vi "error modelling.vi"(10 "Frequency":dbl=200.0, 11 "Gyroscope":dbl[](array[numeric])) -> (1 "actual sample time (s)":dbl)   [LabVIEW 2021]
uses:
  <vilib>/Utility/error.llb/DialogType.ctl
panel:
  out "Allan Variance":dbl
  in  "n":i32
  out "error out 2":errorcluster
  in  "error in (no error) 2":errorcluster
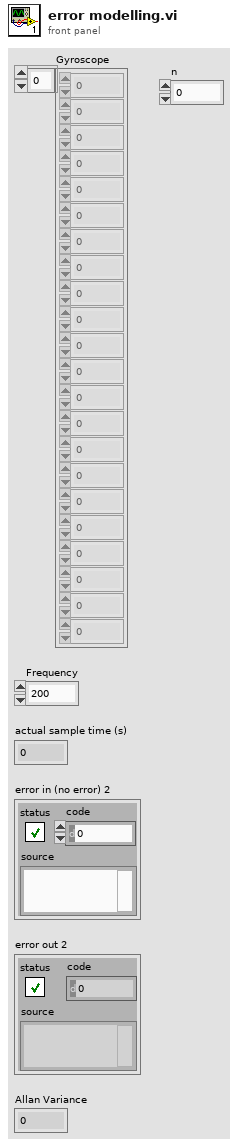
[diagram p1: front panel]
types:
  T1 = typedef "DialogType.ctl" = u16
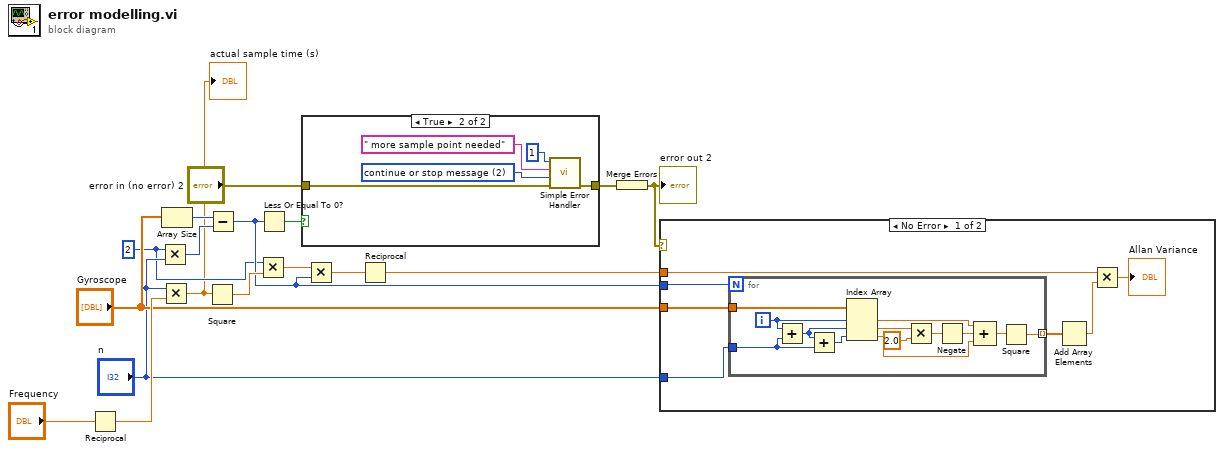
[diagram p0: block diagram]
diagram:
  w3 = 2 ("x")
  n1 = Reciprocal(x="Frequency") -> (1/x=w12:dbl)
  n2 = Multiply(x=w3, y="n") -> (x*y=w10:i32)
  n3 = Multiply(x="n", y=w12) -> (x*y=w1:dbl)
  "actual sample time (s)" <- w1
  n4 = Array Size(array="Gyroscope") -> (size(s)=w11:i32)
  n5 = Square(x=w1) -> (x^2=w9:dbl)
  n6 = Subtract(x=w11, y=w10) -> (x-y=w7:i32)
  n7 = Multiply(x=w3, y=w9) -> (x*y=w8:dbl)
  n8 = Less Or Equal To 0?(x=w7) -> (x <= 0?=w17:bool)
  n9 = case shown="True" w17 {
    tunnel: "error in (no error) 2" -> [w18 w23]
    tunnel: [w18 w22] -> w16
    frame False {
    }
    frame True {
      w20 = T1 2 items=["no dialog", "OK message", "continue or stop message", "OK message + warnings", "continue/stop + warnings"] ("type of dialog (OK msg:1)")
      n10 = call <vilib>:"Simple Error Handler.vi"("error code (no error:0)"=1, "error source (\" \")"=" more sample point needed" ("error source (\" \")"), "type of dialog (OK msg:1)"=w20, "error in (no error)"=w23) -> ("error out"=w22:errorcluster)  [unwired: 1 in, 4 out]
    }
  }
  n11 = Multiply(x=w8, y=w7) -> (x*y=w6:dbl)
  n12 = Reciprocal(x=w6) -> (1/x=w2:dbl)
  n13 = Merge Errors(w16) -> (w14:errorcluster)
  "error out 2" <- w14
  n14 = case shown="No Error" w14 {
    tunnel: w7 -> [w30 _]
    tunnel: "Gyroscope" -> [w29 _]
    tunnel: "n" -> [w28 _]
    tunnel: w2 -> [w25 _]
    frame No Error {
      n15 = for {
        N: w30 -> [_]
        tunnel: w29 -> [w38]
        tunnel: w28 -> [w40]
        tunnel: [w31] -> w27 mode=indexing
        i -> [w41]
        n16 = Add(x=w41, y=w40) -> (x+y=w42:i32)
        n17 = Add(x=w42, y=w40) -> (x+y=w43:i32)
        n18 = Index Array(array=w38, index #1=w41, index #2=w42, index #3=w43) -> (element #1=w39:dbl, element #2=w37:dbl, element #3=w36:dbl)
        n19 = Multiply(x=w37, y=2.0) -> (x*y=w35:dbl)
        n20 = Negate(x=w35) -> (-x=w33:dbl)
        n21 = Compound Arithmetic op=ADD(w39, w33, w36) -> (w32:dbl)
        n22 = Square(x=w32) -> (x^2=w31:dbl)
      }
      n23 = Add Array Elements(numeric array=w27) -> (sum=w26:dbl)
      n24 = Multiply(x=w25, y=w26) -> (x*y=→"Allan Variance":dbl)
    }
    frame Error {
    }
  }
